vi "init_instruments.vi"(10 "LED PSU resource name":refnum<visa-resource-name>="COM6", 11 "SMU resource name":refnum<visa-resource-name>) -> (0 "LED power supply":bool, 1 "Pixel Selector":bool, 4 "SMU":bool)   [LabVIEW 2018]
uses:
  <vilib>/Instr/_visa.llb/VISA Configure Serial Port (Instr).vi
  <instrlib>/Keithley 24XX/Keithley 24XX.lvlib
panel:
  out "TTi power supply":refnum<visa-resource-name>
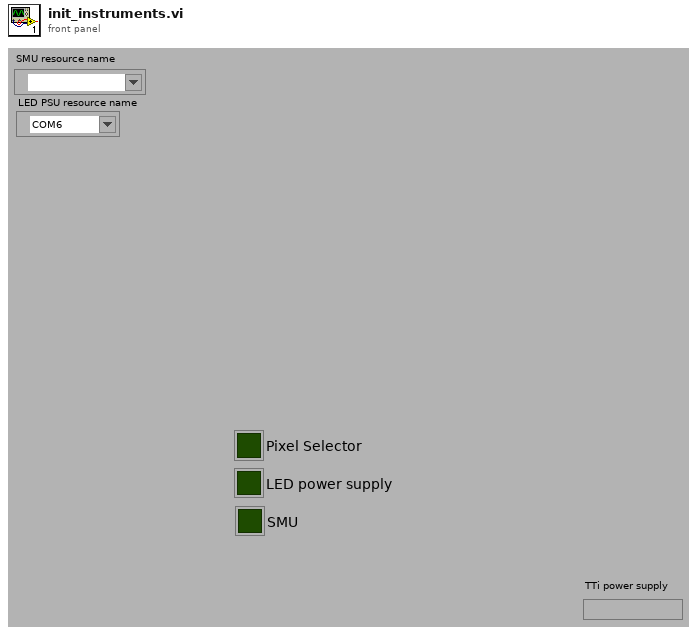
[diagram p1: front panel]
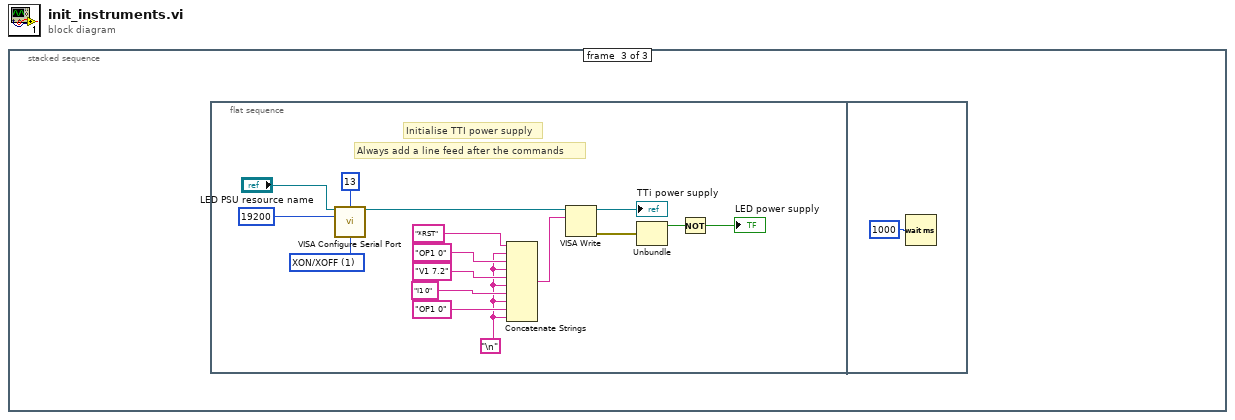
[diagram p0: block diagram]
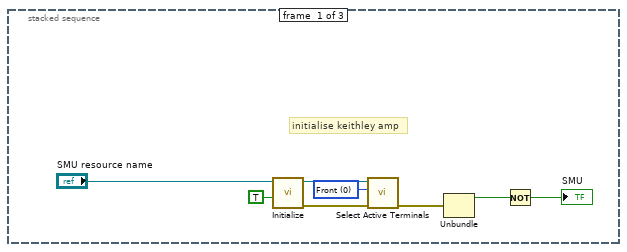
[diagram p2: hidden frame]
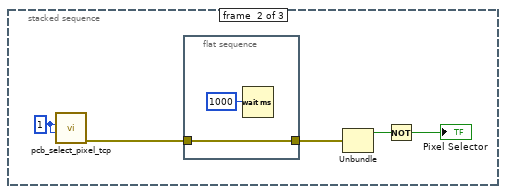
[diagram p3: hidden frame]
diagram:
  n1 = stacked-sequence {
    frame #0 {
      w2 = u16 0 items=["Front", "Rear"] ("Active Terminals (0: Front)")
      # "initialise keithley amp"
      n2 = call <instrlib>:"Initialize.vi"("Reset (True)"=TRUE, "VISA resource name"="SMU resource name") -> ("error out"=w4:errorcluster, "VISA resource name out"=w5:refnum<visa-resource-name>)  [unwired: 8 in]
      n3 = call <instrlib>:"Select Active Terminals.vi"("error in (no error)"=w4, "Active Terminals (0: Front)"=w2, "VISA resource name"=w5) -> ("error out"=w3:errorcluster)  [unwired: 7 in, 1 out]
      n4 = Unbundle(w3) -> ("status"=w8:bool)  [unwired: 2 out]
      n5 = Not(x=w8) -> (.not. x?=→"SMU":bool)
    }
    frame #1 {
      w13 = u32 1 ("Pixel")
      n6 = call "pcb_select_pixel_tcp.vi"("Cell"=w13, "Pixel"=w13) -> ("error out"=w12:errorcluster)  [unwired: 8 in, 1 out]
      n7 = flat-sequence {
        tunnel: w12 -> [w14]
        tunnel: [w14] -> w11
        frame #0 {
          n8 = Wait (ms)(milliseconds to wait=i16 1000 ("Spectrometer Handle in")) -> ()  [unwired: 1 out]
        }
      }
      n9 = Unbundle(w11) -> ("status"=w10:bool)  [unwired: 2 out]
      n10 = Not(x=w10) -> (.not. x?=→"Pixel Selector":bool)
    }
    frame #2 {
      n11 = flat-sequence {
        frame #0 {
          w20 = "\n"
          w27 = u16 1 items=["None", "XON/XOFF", "RTS/CTS", "XON/XOFF & RTS/CTS", "DTR/DSR", "XON/XOFF & DTR/DSR"] ("flow control (0:none)")
          # "Initialise TTI power supply"
          # "Always add a line feed after the commands"
          n12 = call-poly "VISA Configure Serial Port"("VISA resource name"="LED PSU resource name", "termination char\n(0xA = '\\n' = LF)"=u8 13 ("termination char\n(0xA = '\\n' = LF)"), "baud rate (9600)"=u32 19200, "flow control (0:none)"=w27) -> ("VISA resource name out"=w18:refnum<visa-resource-name>)  [unwired: 10 in, 1 out]
          n13 = Concatenate Strings("*RST" ("string"), w20, "OP1 0" ("string"), w20, "V1 7.2" ("string"), w20, "I1 0" ("string"), w20, "OP1 0" ("string"), w20) -> (w19:string)
          n14 = VISA Write(VISA resource name=w18, write buffer=w19) -> (VISA resource name out=→"TTi power supply":refnum<visa-resource-name>, error out=w31:errorcluster)  [unwired: 1 in, 1 out]
          n15 = Unbundle(w31) -> ("status"=w16:bool)  [unwired: 2 out]
          n16 = Not(x=w16) -> (.not. x?=→"LED power supply":bool)
        }
        frame #1 {
          n17 = Wait (ms)(milliseconds to wait=i16 1000 ("Spectrometer Handle in")) -> ()  [unwired: 1 out]
        }
      }
    }
  }
